vi "Hardware Device Get Info.vi"(8 "error in":errorcluster, 11 "NI Analog Input in":refnum<class "NI Analog Input.lvclass">) -> (0 "error out":errorcluster, 3 "NI Analog Input out":refnum<class "NI Analog Input.lvclass">)   [LabVIEW 2023, in "HardwareAbstractionLayer_LVOOP.lvlib" / "NI Analog Input.lvclass"]
doc: "This VI is AI Physical Channel Read"
uses:
  NI Analog Input.lvclass
  NI Analog Input.lvclass/NI Analog Input.ctl
  <resource>/objmgr/daqmx.rc
  Teststand/Teststand.lvclass
panel:
  out "AI.PhysicalChans":tag[](array[tag])
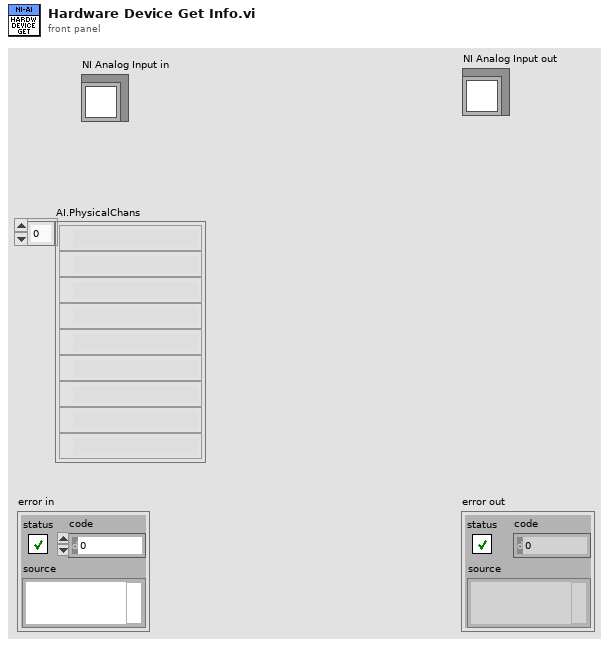
[diagram p1: front panel]
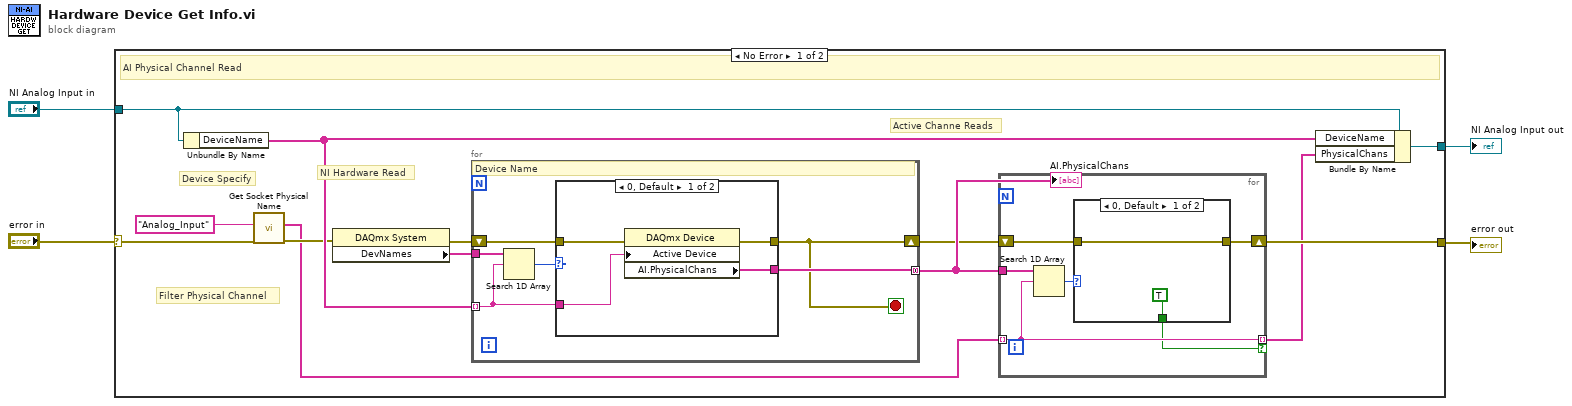
[diagram p0: block diagram]
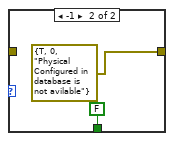
[diagram p2: hidden frame]
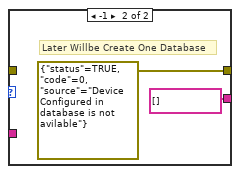
[diagram p3: hidden frame]
diagram:
  n1 = case shown="No Error" "error in" {
    selector: "error in" -> [w8 w41]
    tunnel: [w10 w41] -> w3
    tunnel: [w17 w40] -> w1
    tunnel: "NI Analog Input in" -> [w16 w40]
    frame No Error {
      # "Filter Physical Channel"
      # "Active Channe Reads"
      # "Device Specify"
      # "NI Hardware Read"
      # "AI Physical Channel Read"
      n2 = Unbundle By Name(w16) -> ("DeviceName"=w15:tag[])
      n3 = call "Get Socket Physical Name.vi"("error In"=w8, "ChannelType"="Analog_Input") -> ("error out"=w7:errorcluster, "Physical Channel"=w5:tag[])  [unwired: 7 in, 1 out]
      n4 = property class="DAQmx System"(error in=w7) -> (error out=w13:errorcluster, "DevNames"=w14:tag[])  [unwired: 1 in, 1 out]
      n5 = for {
        tunnel: w15 -> [w30] mode=indexing
        tunnel: w14 -> [w31]
        tunnel: [w29] -> w12 mode=concatenating
        shift-right: [w28] -> w11
        shift-left: w13 -> [w32]
        stop <- w28 stop-if-true
        # "Device Name"
        n6 = Search 1D Array(1D array=w31, element=w30) -> (index of element=w33:i32)  [unwired: 1 in]
        n7 = case shown="0, Default" w33 {
          tunnel: w32 -> [w35 _]
          tunnel: [w34 errorcluster {"status"=TRUE, "code"=0, "source"="Device  Configured in database is not avilable"} ("error out")] -> w28
          tunnel: w30 -> [w37 _]
          tunnel: [w36 tag[] [] ("AI.PhysicalChans")] -> w29
          frame 0, Default {
            n8 = property class="DAQmx Device"(error in=w35, "Active Device"=w37) -> (error out=w34:errorcluster, "AI.PhysicalChans"=w36:tag[])  [unwired: 1 in, 1 out]
          }
          frame -1 {
            # "Later Willbe Create One Database"
          }
        }
      }
      "AI.PhysicalChans" <- w12
      n9 = for {
        tunnel: w12 -> [w23]
        tunnel: w5 -> [w19] mode=indexing
        shift-right: [w20] -> w10
        shift-left: w11 -> [w21]
        tunnel: [w19] -> w9 mode=indexing if=w18
        n10 = Search 1D Array(1D array=w23, element=w19) -> (index of element=w22:i32)  [unwired: 1 in]
        n11 = case shown="0, Default" w22 {
          tunnel: w21 -> [w25 _]
          tunnel: [w25 errorcluster {"status"=TRUE, "code"=0, "source"="Physical Configured in database is not avilable"} ("error out")] -> w20
          tunnel: [TRUE FALSE] -> w18
          frame 0, Default {
          }
          frame -1 {
          }
        }
      }
      n12 = Bundle By Name(cluster=w16, "DeviceName"=w15, "PhysicalChans"=w9) -> (w17:refnum<class "NI Analog Input.lvclass">)
    }
    frame Error {
    }
  }
  "error out" <- w3
  "NI Analog Input out" <- w1
